vi "Open_Door_Selection.vi"(8 "error in (no error)":errorcluster, 10 "raw scan code":string, 11 "Cluster In":T1) -> (0 "error out":errorcluster, 2 "String":string, 3 "Cluster Out":T1)   [LabVIEW 2017]
uses:
  Controls/Feed_Cyc_Data.ctl
  Controls/QUEUE_STATES.ctl
  Controls/Feed_St.ctl
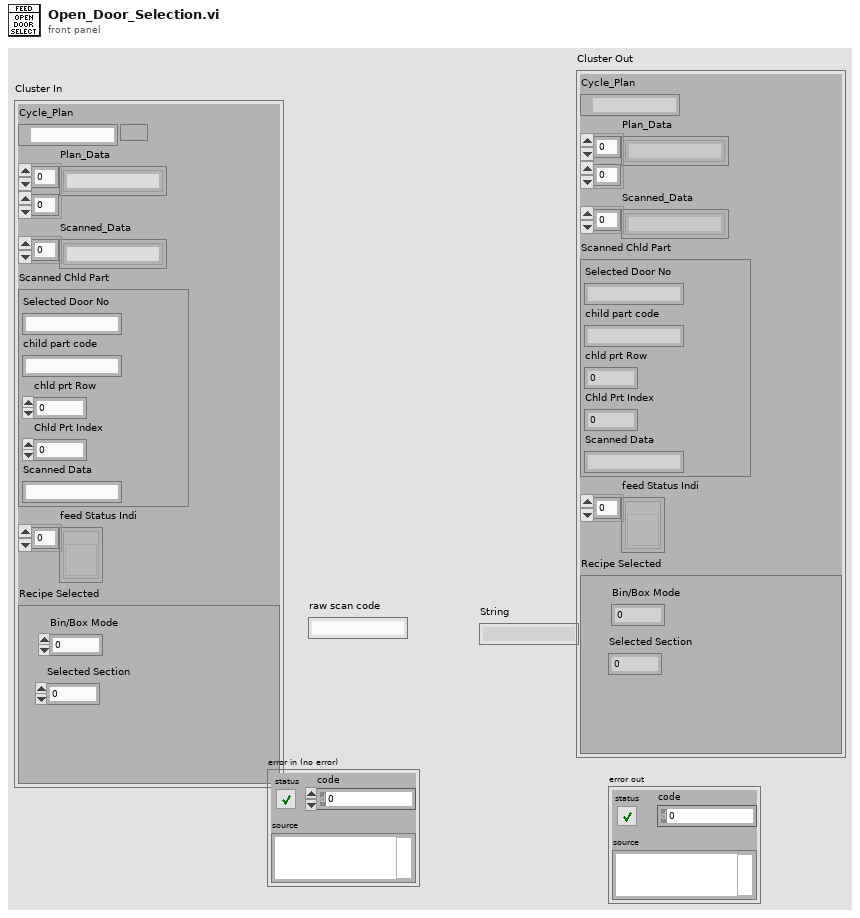
[diagram p1: front panel]
types:
  T1 = typedef "Feed_Cyc_Data.ctl" = cluster{"Cycle_Plan":path, "Plan_Data":string[][], "Scanned_Data":string[], "Scanned Chld Part":cluster{"Selected Door No":string, "child part code":string, "chld prt Row":i32, "Chld Prt Index":i32, "Scanned Data":string}, "feed Status Indi":refnum<vi>[], "Recipe Selected":cluster{"Bin/Box Mode":i32, "Selected Section":i32}}
  T2 = typedef "Feed_St.ctl" = enum16{"Package_Qty_Count", "GENERATE_QR_PRNT", "Cluster_update", "Read_Plan", "QR_Scanned", "Int", "SaveReport ", "Open_Door", "Error_Handler", "Wait", "Close_Door", "Stop"}
  T3 = typedef "QUEUE_STATES.ctl" = enum16{"CREATE Q", "EN Q", "DE Q", "CLOSE Q"}
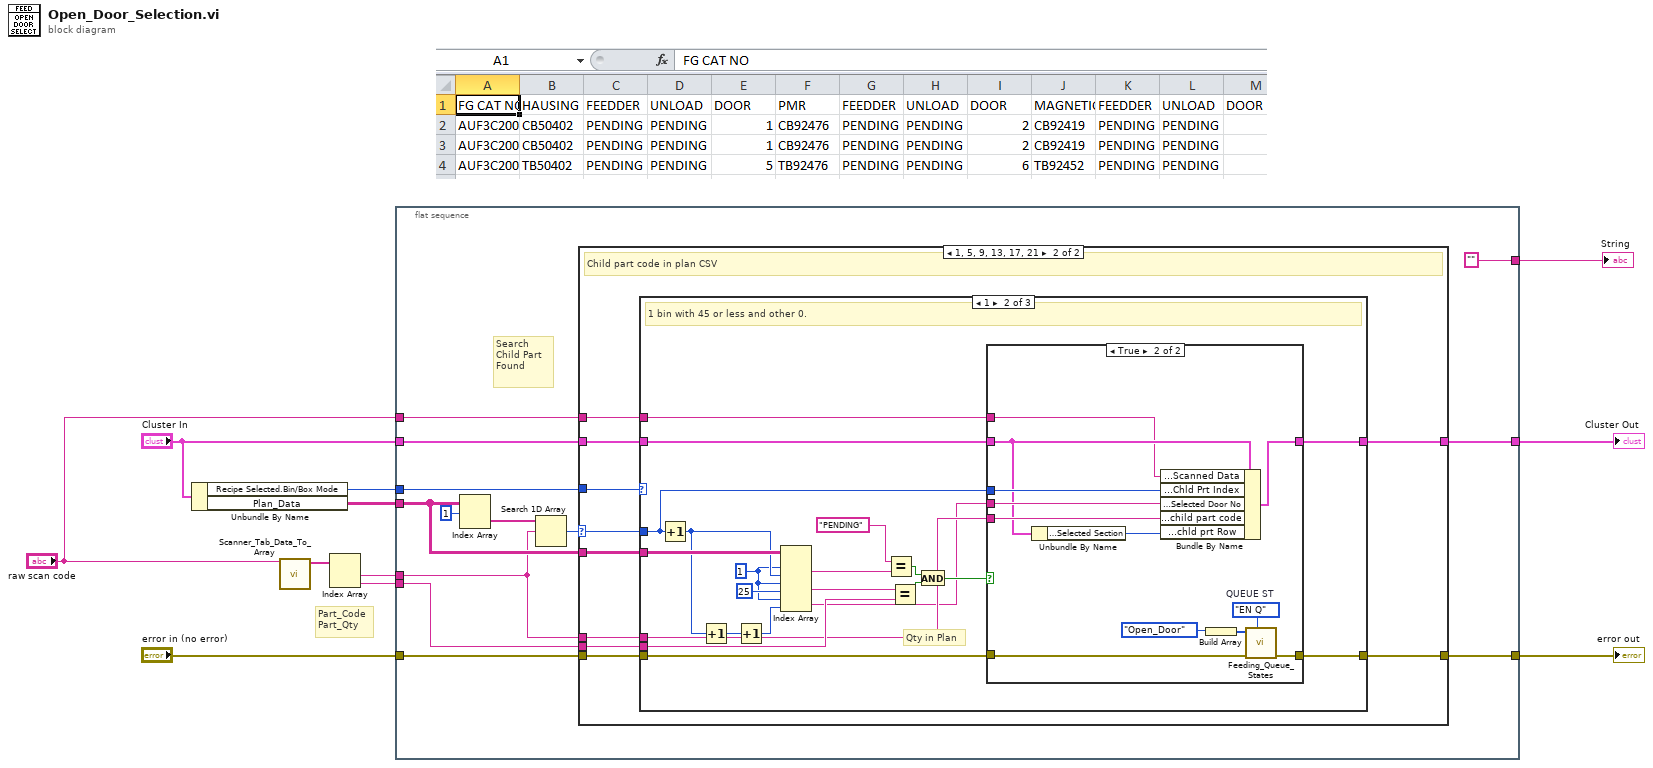
[diagram p0: block diagram]
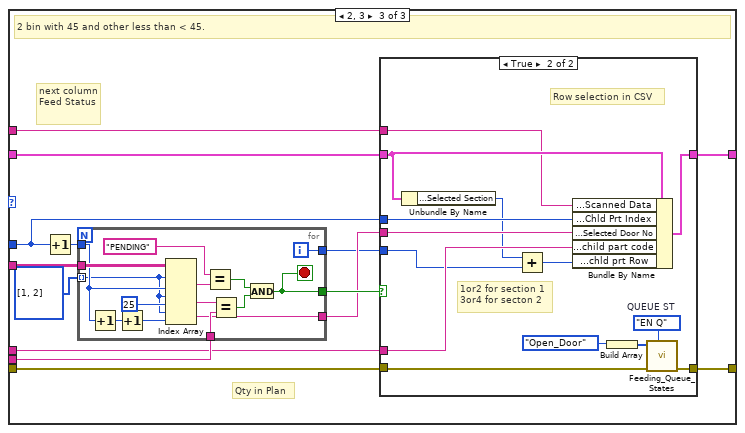
[diagram p5: hidden frame]
diagram:
  # "Part_Code\nPart_Qty"
  n1 = Unbundle By Name("Cluster In") -> ("Recipe Selected.Bin/Box Mode"=w7:i32, "Plan_Data"=w5:string[][])
  n2 = call "Scanner_Tab_Data_To_Array.vi"("Scanner Data"="raw scan code") -> ("Array"=w3:string[])  [unwired: 10 in]
  n3 = Index Array(array=w3) -> (element #1=w6:string, element #2=w10:string)  [unwired: 2 in]
  n4 = flat-sequence {
    tunnel: "error in (no error)" -> [w19]
    tunnel: [w18] -> w4
    tunnel: w5 -> [w20]
    tunnel: w6 -> [w13]
    tunnel: w7 -> [w21]
    tunnel: "Cluster In" -> [w17]
    tunnel: [w16] -> w9
    tunnel: w10 -> [w15]
    tunnel: [""] -> w11
    tunnel: "raw scan code" -> [w12]
    frame #0 {
      # "Search Child Part Found"
      n5 = Index Array(array=w20, index (row)=1) -> (element=w24:string[])  [unwired: 1 in]
      n6 = Search 1D Array(1D array=w24, element=w13) -> (index of element=w22:i32)  [unwired: 1 in]
      n7 = case shown="1, 5, 9, 13, 17, 21" w22 {
        selector: w22 -> [_ w34]
        tunnel: w21 -> [_ w36]
        tunnel: w20 -> [_ w35]
        tunnel: [w26 w33] -> w18
        tunnel: w19 -> [w26 w32]
        tunnel: w17 -> [w25 w31]
        tunnel: [w25 w30] -> w16
        tunnel: w15 -> [_ w29]
        tunnel: w13 -> [_ w28]
        tunnel: w12 -> [_ w27]
        frame -1, Default {
          # "wrong child part/bin part\nscanner"
        }
        frame 1, 5, 9, 13, 17, 21 {
          # "Child part code in plan CSV"
          n8 = case shown="1" w36 {
            tunnel: w35 -> [_ w59 w87]
            tunnel: w34 -> [_ w42 w78]
            tunnel: [w38 w55 w85] -> w33
            tunnel: w32 -> [w38 w56 w86]
            tunnel: w31 -> [w37 w41 w77]
            tunnel: [w37 w54 w84] -> w30
            tunnel: w29 -> [_ w52 w83]
            tunnel: w28 -> [_ w48 w81]
            tunnel: w27 -> [_ w39 w74]
            frame 0, Default {
            }
            frame 1 {
              w40 = 1
              # "Qty in Plan"
              # "1 bin with 45 or less and other 0."
              n9 = Increment(x=w42) -> (x+1=w46:i32)
              n10 = Increment(x=w46) -> (x+1=w45:i32)
              n11 = Increment(x=w45) -> (x+1=w44:i32)
              n12 = Index Array(array=w59, index (row) #1=w40, index (col) #1=w46, index (row) #2=w40, index (col) #2=25, index (row) #3=w40, index (col) #3=w44) -> (element #1=w58:string, element #2=w53:string, element #3=w43:string)
              n13 = Equal?(x="PENDING", y=w58) -> (x = y?=w50:bool)
              n14 = Equal?(x=w53, y=w52) -> (x = y?=w51:bool)
              n15 = And(x=w50, y=w51) -> (x .and. y?=w49:bool)
              n16 = case shown="True" w49 {
                tunnel: w56 -> [w61 w72]
                tunnel: [w61 w71] -> w55
                tunnel: w41 -> [w60 w64]
                tunnel: [w60 w68] -> w54
                tunnel: w48 -> [_ w67]
                tunnel: w43 -> [_ w66]
                tunnel: w42 -> [_ w65]
                tunnel: w39 -> [_ w62]
                frame False {
                }
                frame True {
                  w73 = QUEUE_STATES."EN Q"  # QUEUE ST
                  n17 = Unbundle By Name(w64) -> ("Recipe Selected.Selected Section"=w63:i32)
                  n18 = Bundle By Name(cluster=w64, "Scanned Chld Part.Scanned Data"=w62, "Scanned Chld Part.Chld Prt Index"=w65, "Scanned Chld Part.Selected Door No"=w66, "Scanned Chld Part.child part code"=w67, "Scanned Chld Part.chld prt Row"=w63) -> (w68:T1)
                  n19 = Build Array(Feed_St."Open_Door" ("Feed ST")) -> (w69:T2[])
                  n20 = call "Feeding_Queue_States.vi"("QUEUE ST"=w73, "error in"=w72, "Feed St"=w69) -> ("error OUT"=w71:errorcluster)  [unwired: 7 in, 1 out]
                }
              }
            }
            frame 2, 3 {
              # "next column Feed Status"
              # "Qty in Plan"
              # "2 bin with 45 and other less than < 45."
              n21 = Increment(x=w78) -> (x+1=w80:i32)
              n22 = for {
                tunnel: w87 -> [w102]
                tunnel: w83 -> [w98]
                tunnel: [w89] -> w82
                tunnel: w80 -> [w94]
                tunnel: [w91] -> w79
                tunnel: i32[] [1, 2] -> [w90] mode=indexing
                tunnel: [w88] -> w75
                i -> [w88]
                stop <- w89 stop-if-true
                n23 = Increment(x=w94) -> (x+1=w93:i32)
                n24 = Increment(x=w93) -> (x+1=w92:i32)
                n25 = Index Array(array=w102, index (row) #1=w90, index (col) #1=w94, index (row) #2=w90, index (col) #2=25, index (row) #3=w90, index (col) #3=w92) -> (element #1=w101:string, element #2=w99:string, element #3=w91:string)
                n26 = Equal?(x="PENDING", y=w101) -> (x = y?=w96:bool)
                n27 = Equal?(x=w99, y=w98) -> (x = y?=w97:bool)
                n28 = And(x=w96, y=w97) -> (x .and. y?=w89:bool)
              }
              n29 = case shown="True" w82 {
                tunnel: w86 -> [w104 w117]
                tunnel: [w104 w116] -> w85
                tunnel: w77 -> [w103 w109]
                tunnel: [w103 w113] -> w84
                tunnel: w81 -> [_ w112]
                tunnel: w79 -> [_ w111]
                tunnel: w78 -> [_ w110]
                tunnel: w75 -> [_ w106]
                tunnel: w74 -> [_ w105]
                frame False {
                }
                frame True {
                  w118 = QUEUE_STATES."EN Q"  # QUEUE ST
                  # "1or2 for section 1\n3or4 for secton 2"
                  # "Row selection in CSV"
                  n30 = Unbundle By Name(w109) -> ("Recipe Selected.Selected Section"=w107:i32)
                  n31 = Add(x=w107, y=w106) -> (x+y=w108:i32)
                  n32 = Bundle By Name(cluster=w109, "Scanned Chld Part.Scanned Data"=w105, "Scanned Chld Part.Chld Prt Index"=w110, "Scanned Chld Part.Selected Door No"=w111, "Scanned Chld Part.child part code"=w112, "Scanned Chld Part.chld prt Row"=w108) -> (w113:T1)
                  n33 = Build Array(Feed_St."Open_Door" ("Feed ST")) -> (w114:T2[])
                  n34 = call "Feeding_Queue_States.vi"("QUEUE ST"=w118, "error in"=w117, "Feed St"=w114) -> ("error OUT"=w116:errorcluster)  [unwired: 7 in, 1 out]
                }
              }
            }
          }
        }
      }
    }
  }
  "String" <- w11
  "Cluster Out" <- w9
  "error out" <- w4
